vi "Close Nitro Valve.vi"(8 "error in (no error)":errorcluster, 11 "FPGA API Concrete in":refnum<class "FPGA API Concrete.lvclass">) -> (0 "error out":errorcluster, 3 "FPGA API Concrete out":refnum<class "FPGA API Concrete.lvclass">)   [LabVIEW 2019, in "FPGA API Concrete.lvclass"]
uses:
  FPGA API Concrete.lvclass
  D:/GIT H4000/H4000/src/FPGA_API_class/FPGA API.lvclass
  FPGA_API_class/FPGA API.lvclass/FPGA API.ctl
  FPGA API Concrete.lvclass/FPGA API Concrete.ctl
  <vilib>/Utility/error.llb/Error Cluster From Error Code.vi
  <vilib>/rvi/errors/niLvFpgaAdjustHostInterfaceError.vi
  <vilib>/rvi/interface/nirviMethod/nirviMethod.xnode
  FPGA Ref.ctl
  FPGA_API_class/FPGA API.lvclass
  <vilib>/FPGAPlugInAG/Dynamic/niLvFpga_WriteFifo_Dynamic.vi
  <vilib>/rvi/errors/niLvFpgaMergeErrorWithErrorCode.vi
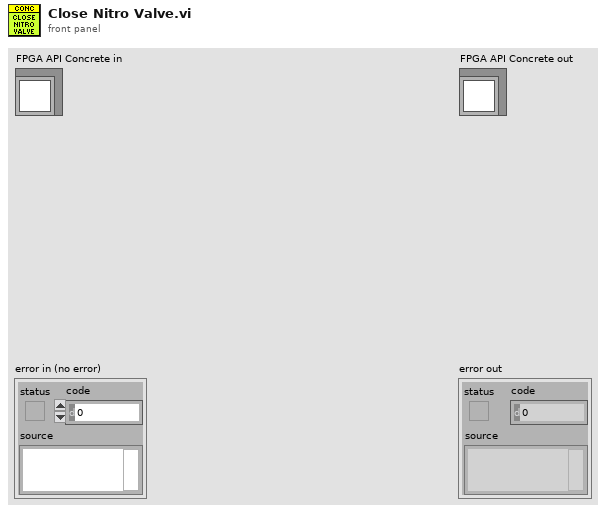
[diagram p1: front panel]
types:
  T1 = typedef "DO index.ctl" = u8
  T2 = typedef "FPGA API Concrete.lvclass/FPGA Ref.ctl" = refnum<k20>
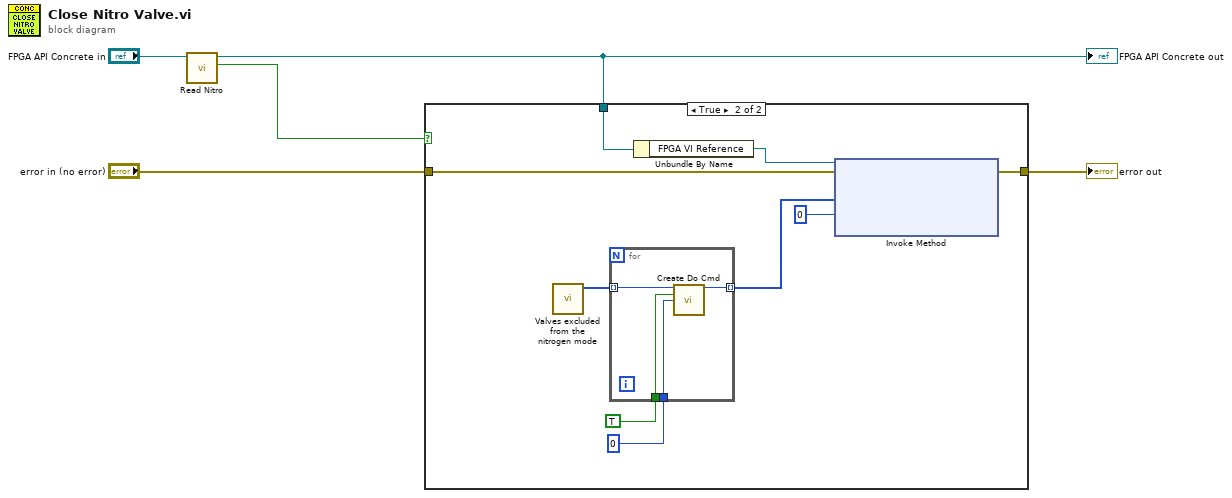
[diagram p0: block diagram]
diagram:
  n1 = call "Read Nitro.vi"("FPGA API in"="FPGA API Concrete in") -> ("Nitro"=w1:bool, "FPGA API out"=w3:refnum<class "FPGA API Concrete.lvclass">)  [unwired: 9 in]
  "FPGA API Concrete out" <- w3
  n2 = case shown="True" w1 {
    tunnel: "error in (no error)" -> [w6 w13]
    tunnel: [w6 w12] -> w2
    tunnel: w3 -> [_ w11]
    frame False {
    }
    frame True {
      n3 = call "Valves excluded from the nitrogen mode.vi"() -> ("#DO"=w7:T1[])  [unwired: 11 in]
      n4 = for {
        tunnel: w7 -> [w19] mode=indexing
        tunnel: [w18] -> w10 mode=indexing
        tunnel: u32 0 ("Time uSec") -> [w17]
        tunnel: TRUE ("value") -> [w16]
        n5 = call "Create Do Cmd.vi"("#DO"=w19, "value"=w16, "Time uSec"=w17) -> ("Numeric"=w18:u64)  [unwired: 12 in]
      }
      n6 = Unbundle By Name(w11) -> ("FPGA VI Reference"=w14:T2)
      n7 = xnode "Invoke Method"("FPGA VI Reference In"=w14, "error in"=w13, "Data"=w10, "Timeout (ms)"=0) -> ("error out"=w12:errorcluster)  [unwired: 2 out]
    }
  }
  "error out" <- w2
